vi "Send Launch Measurements Message.vi"(6 "Show FP?":bool, 8 "error in (no error)":errorcluster, 9 "Device Names":string[](array[string]), 10 "Measurement Name":string, 11 "Self Enqueuer In":refnum<class "Message Enqueuer.lvclass">) -> (0 "error out":errorcluster, 3 "Self Enqueuer Out":refnum<class "Message Enqueuer.lvclass">)   [LabVIEW 2015, in "Controller Actor.lvlib" / "Launch Measurements Message.lvclass"]
uses:
  Launch Measurements Message.lvclass
  <vilib>/ActorFramework/Message Enqueuer/Message Enqueuer.lvclass
  Launch Measurements Message.lvclass/Launch Measurements Message.ctl
  <vilib>/ActorFramework/Message Enqueuer/Message Enqueuer.lvclass/Message Enqueuer.ctl
  <vilib>/ActorFramework/Message Priority Queue/Priority Enqueue.vi
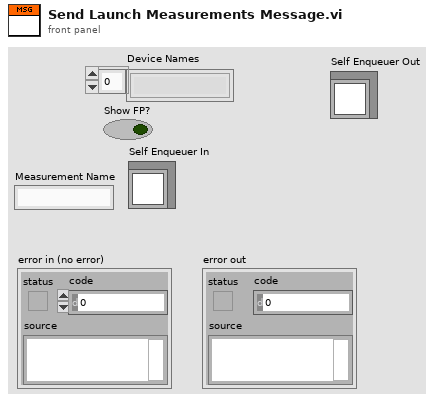
[diagram p1: front panel]
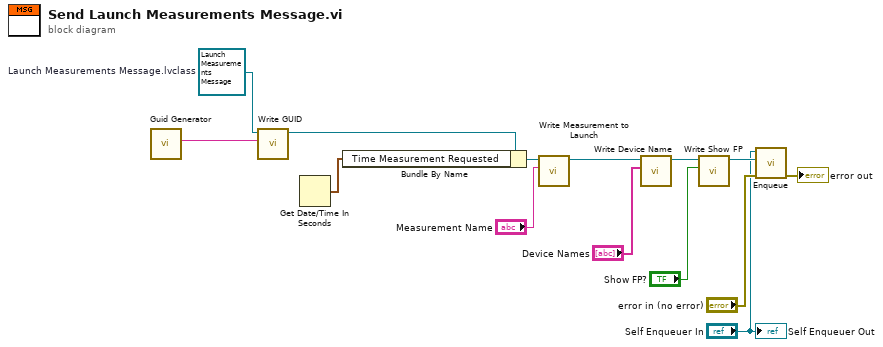
[diagram p0: block diagram]
diagram:
  w5 = refnum<class "Launch Measurements Message.lvclass"> refnum  # Launch Measurements Message.lvclass
  n1 = call <vilib>:"Guid Generator.vi"() -> ("GUID"=w1:string)  [unwired: 10 in, 1 out]
  n2 = call "Write GUID.vi"("GUID"=w1, "Launch Measurements Message in"=w5) -> ("Launch Measurements Message out"=w2:refnum<class "Launch Measurements Message.lvclass">)  [unwired: 8 in, 1 out]
  n3 = Get Date/Time In Seconds() -> (seconds since 1Jan1904=w3:timestamp)
  n4 = Bundle By Name(cluster=w2, "Time Measurement Requested"=w3) -> (w4:refnum<class "Launch Measurements Message.lvclass">)
  n5 = call "Write Measurement to Launch.vi"("Measurement Name"="Measurement Name", "Launch Measurements Message in"=w4) -> ("Launch Measurements Message out"=w13:refnum<class "Launch Measurements Message.lvclass">)  [unwired: 8 in, 1 out]
  n6 = call "Write Device Name.vi"("Device Names"="Device Names", "Launch Measurements Message in"=w13) -> ("Launch Measurements Message out"=w10:refnum<class "Launch Measurements Message.lvclass">)  [unwired: 8 in, 1 out]
  n7 = call "Write Show FP.vi"("Show FP?"="Show FP?", "Launch Measurements Message in"=w10) -> ("Launch Measurements Message out"=w9:refnum<class "Launch Measurements Message.lvclass">)  [unwired: 8 in, 1 out]
  n8 = call <vilib>:"Enqueue.vi"("error in (no error)"="error in (no error)", "Message"=w9, "Message Enqueuer in"="Self Enqueuer In") -> ("error out"=→"error out":errorcluster)  [unwired: 7 in, 1 out]
  "Self Enqueuer Out" <- "Self Enqueuer In"
